vi "Configure Channels.vi"(8 "error in (no error)":errorcluster, 11 "DI DAQmx CFG in":refnum<class "DI DAQmx CFG.lvclass">) -> (0 "error out":errorcluster, 3 "DI DAQmx CFG out":refnum<class "DI DAQmx CFG.lvclass">)   [LabVIEW 2023, in "DI DAQmx CFG.lvclass"]
uses:
  DI DAQmx CFG.lvclass
  Configuration/Configuration JSON/Configuration JSON Base/CFG JSON.lvclass/CFG JSON.ctl
  DAQmx/DAQmx Base CFG/DAQmx Base CFG.lvclass/DAQmx Base CFG.ctl
  837b5ed5-0c17-42a6-9ee3-103f8da6f62b.vi
  <vilib>/JDP Science/JSONtext/Find Item.vi
  <vilib>/JDP Science/JSONtext/Next JSON Value.vi
  <vilib>/JDP Science/JSONtext/String Subset.vi
  <vilib>/JDP Science/JSONtext/Parsing/Advance past next JSON Value (inlined COPY).vi
  <vilib>/JDP Science/JSONtext/Parsing/Advance past whitespace.vi
  <vilib>/JDP Science/JSONtext/Parsing/Advance past String.vi
  <vilib>/JDP Science/JSONtext/Parsing/Advance past Number.vi
  <vilib>/JDP Science/JSONtext/Parsing/Advance past Line Ending.vi
  <vilib>/JDP Science/JSONtext/Parsing/Parse Full Path or Item Name.vi
  <vilib>/JDP Science/JSONtext/Parsing/Advance past Array.vi
  <vilib>/JDP Science/JSONtext/Parsing/Advance past Object.vi
  <vilib>/JDP Science/JSONtext/support/Error Cluster From Code.vi
  <vilib>/JDP Science/JSONtext/Offset/Find Item Locations by Path.vi
  <vilib>/JDP Science/JSONtext/JSON text to Variant.vi
  <vilib>/Utility/error.llb/Error Cluster From Error Code.vi
  <vilib>/DAQmx/create/channels.llb/DAQmx Create Channel (DI-Digital Input).vi
  <vilib>/JDP Science/JSONtext/LVClass Serializer/JSONtext LVClass Serializer.lvclass
  <vilib>/ErrorRing/Error Ring.xnode
  DI DAQmx CFG.lvclass/DI DAQmx CFG.ctl
  DAQmx/DAQmx Base CFG/DAQmx Base CFG.lvclass
  Configuration/Configuration JSON/Configuration JSON Base/CFG JSON.lvclass
panel:
  out "Line Grouping":i32(ring)=1 items=["one channel for each line", "one channel for all lines"]
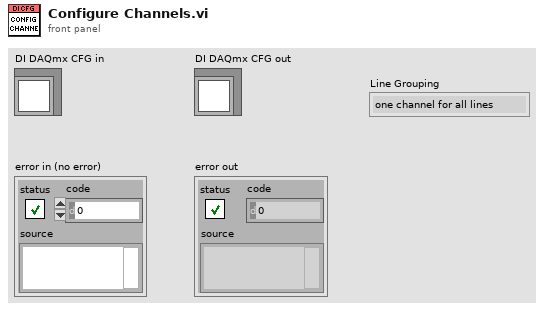
[diagram p1: front panel]
types:
  T1 = cluster{"Name":string, "Enabled":bool, "Line Grouping":string, "Port":string}[]
  T2 = typedef "LVStringsAndValuesArrayTypeDef_I32.ctl" = cluster{"String":string, "Value":i32}[]
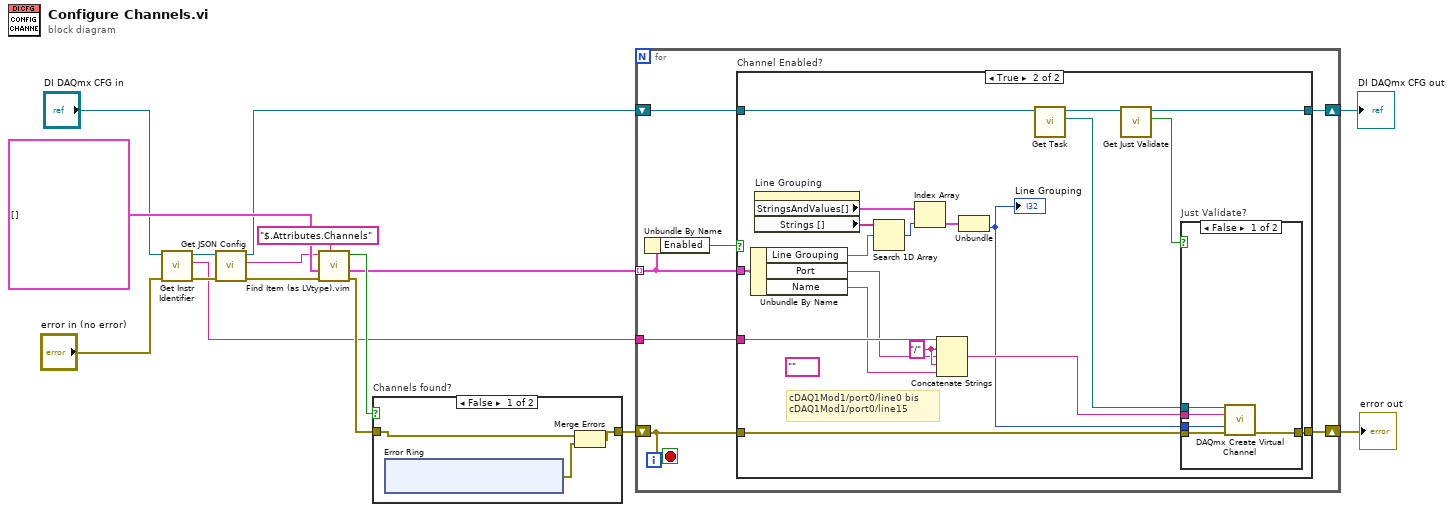
[diagram p0: block diagram]
diagram:
  n1 = call-dynamic "Get Instr Identifier.vi"("error in (no error)"="error in (no error)", "Configuration Base in"="DI DAQmx CFG in") -> ("error out"=w8:errorcluster, "Instr Identifier"=w6:string, "Configuration Base out"=w7:refnum<class "DI DAQmx CFG.lvclass">)  [unwired: 7 in]
  n2 = call "Get JSON Config.vi"("error in (no error)"=w8, "CFG Base in"=w7) -> ("error out"=w15:errorcluster, "<JSON>Config>"=w9:string, "CFG Base out"=w5:refnum<class "DI DAQmx CFG.lvclass">)  [unwired: 7 in]
  n3 = call "Find Item (as LVtype).vim"("$Path or Item Name"="$.Attributes.Channels", "error in (no error)"=w15, "Data Type and Default Value"=T1 [], "JSON"=w9) -> ("error out"=w13:errorcluster, "Data"=w11:T1, "Found"=w14:bool)  [unwired: 4 in, 1 out]
  n4 = case "Channels found?" shown="False" w14 {
    tunnel: w13 -> [w19 w25]
    tunnel: [w17 w25] -> w12
    frame False {
      n5 = xnode "Error Ring"() -> ("error out"=w18:errorcluster)
      n6 = Merge Errors(w19, w18) -> (w17:errorcluster)
    }
    frame True {
    }
  }
  n7 = for {
    tunnel: w11 -> [w29] mode=indexing
    shift-right: [w32] -> w1
    shift-left: w12 -> [w31]
    tunnel: w6 -> [w30]
    shift-right: [w27] -> w2
    shift-left: w5 -> [w26]
    stop <- w31 stop-if-true
    n8 = Unbundle By Name(w29) -> ("Enabled"=w28:bool)
    n9 = case "Channel Enabled?" shown="True" w28 {
      tunnel: [w34 w43] -> w32
      tunnel: w31 -> [w34 w51]
      tunnel: w30 -> [_ w50]
      tunnel: w29 -> [_ w49]
      tunnel: [w33 w40] -> w27
      tunnel: w26 -> [w33 w41]
      frame False {
      }
      frame True {
        (unwired) tag "" ("DAQmx Physical Channel")
        w38 = "/" ("string")
        # "cDAQ1Mod1/port0/line0 bis\ncDAQ1Mod1/port0/line15"
        n10 = Unbundle By Name(w49) -> ("Line Grouping"=w45:string, "Port"=w37:string, "Name"=w36:string)
        n11 = property on="Line Grouping" class="Ring (strict)"() -> ("StringsAndValues[]"=w53:T2, "Strings []"=w47:string[])  [unwired: 2 in, 2 out]
        n12 = Search 1D Array(1D array=w47, element=w45) -> (index of element=w46:i32)  [unwired: 1 in]
        n13 = Index Array(array=w53, index=w46) -> (element=w52:cluster{"String":string, "Value":i32})
        n14 = Concatenate Strings(w50, w38, w37, w38, w36) -> (w48:string)
        n15 = Unbundle(w52) -> ("Value"=w35:i32)  [unwired: 1 out]
        "Line Grouping" <- w35
        n16 = call "Get Task.vi"("DAQmx Base CFG in"=w41) -> ("Task"=w44:refnum<k21>, "DAQmx Base CFG out"=w42:refnum<class "DI DAQmx CFG.lvclass">)  [unwired: 8 in, 1 out]
        n17 = call "Get Just Validate.vi"("CFG JSON Base in"=w42) -> ("Just Validate"=w39:bool, "CFG JSON Base out"=w40:refnum<class "DI DAQmx CFG.lvclass">)  [unwired: 8 in, 1 out]
        n18 = case "Just Validate?" shown="False" w39 {
          tunnel: w51 -> [w58 w59]
          tunnel: w48 -> [w55 _]
          tunnel: w44 -> [w57 _]
          tunnel: [w56 w59] -> w43
          tunnel: w35 -> [w54 _]
          frame False {
            n19 = call-poly <vilib>:"DAQmx Create Virtual Channel.vi"("task in"=w57, "lines"=w55, "line grouping"=w54, "error in"=w58) -> ("error out"=w56:errorcluster)  [unwired: 10 in, 1 out]
          }
          frame True {
          }
        }
      }
    }
  }
  "error out" <- w1
  "DI DAQmx CFG out" <- w2
